vi "temperature header.vi"() -> (0 "Array":string[][](array[string]))   [LabVIEW 2021]
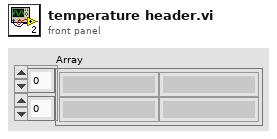
[diagram p1: front panel]
types:
  T1 = enum16{"pot_temp", "sorb_temp", "needle_valve_temp", "still_temp", "mix_chamber_temp", "stm_rx_temp", "stm_cx_temp", "tank_pressure", "condense_pressure", "still_pressure", "turbo_back_pressure", "n2_trap_pressure"}
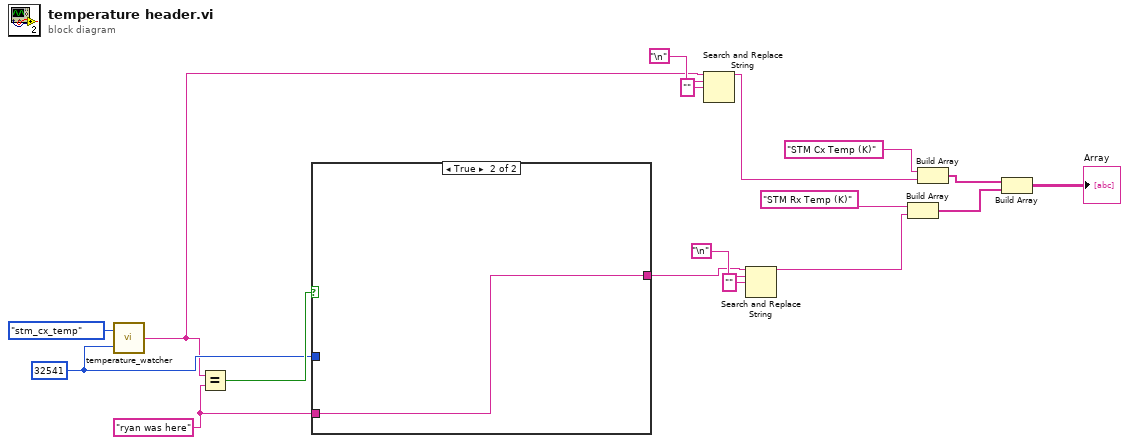
[diagram p0: block diagram]
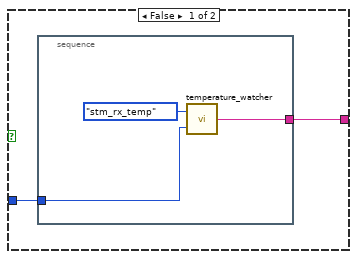
[diagram p2: hidden frame]
diagram:
  w9 = u16 32541 ("Port Number")
  w11 = "ryan was here"
  n1 = call "temperature_watcher.vi"("Port Number"=w9, "Command"=T1."stm_cx_temp") -> ("Response"=w6:string)
  n2 = Equal?(x=w6, y=w11) -> (x = y?=w12:bool)
  n3 = case shown="True" w12 {
    tunnel: w11 -> [_ w23]
    tunnel: w9 -> [w19 _]
    tunnel: [w18 w23] -> w2
    frame False {
      n4 = stacked-sequence {
        tunnel: w19 -> [w22]
        tunnel: [w20] -> w18
        frame #0 {
          n5 = call "temperature_watcher.vi"("Port Number"=w22, "Command"=T1."stm_rx_temp") -> ("Response"=w20:string)
        }
      }
    }
    frame True {
    }
  }
  n6 = Search and Replace String(input string=w6, search string="\n", replace string="" ("replace string (\"\")")) -> (result string=w5:string)  [unwired: 5 in, 3 out]
  n7 = Search and Replace String(input string=w2, search string="\n", replace string="" ("replace string (\"\")")) -> (result string=w1:string)  [unwired: 5 in, 3 out]
  n8 = Build Array("STM Rx Temp (K)", w1) -> (w13:string[])
  n9 = Build Array("STM Cx Temp (K)", w5) -> (w16:string[])
  n10 = Build Array(w16, w13) -> (→"Array":string[][])
